vi "0xE7_Read_description_one_float_parameter.vi"(8 "error in":errorcluster, 10 "NumberFloatParam":i32 format="%0d", 11 "paramUnicornIn in":T2) -> (0 "error out":errorcluster, 1 "Param":T1, 2 "Тип/версия устройства":string, 3 "paramUnicornIn out 2":T2)   [LabVIEW 2017, in "LV_Unicorn.lvlib"]
uses:
  LV_Unicorn.lvlib
  Control/unicorn_Param.ctl
  Control/unicorn_conn.ctl
  Control/unicorn_JSON.ctl
  Control/unicorn_ParamInt.ctl
  Control/unicorn_Telemetry.ctl
  Control/unicorn_Table.ctl
  Control/unicorn_ParamFloat.ctl
  Control/unicorn_DescriptParam.ctl
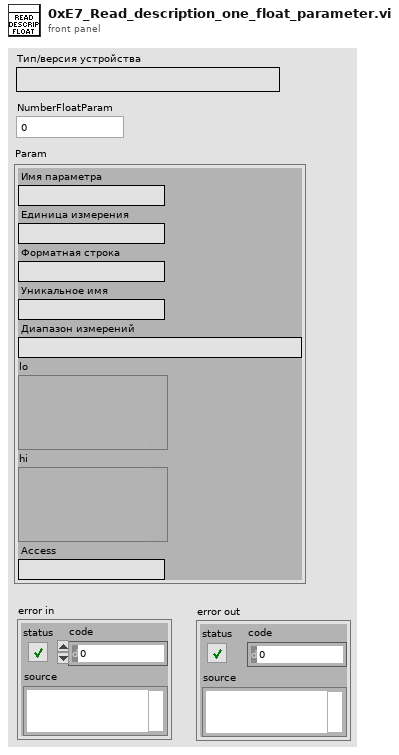
[diagram p1: front panel]
types:
  T1 = typedef "unicorn_DescriptParam.ctl" = cluster{"Имя параметра":string, "Единица измерения":string, "Форматная строка ":string, "Уникальное имя":string, "Диапазон измерений":string, "lo":variant, "hi":variant, "Access":string}
  T2 = typedef "LV_Unicorn.lvlib/unicorn_Param.ctl" = cluster{"conParam":T3, "Param":T4}
  T3 = typedef "LV_Unicorn.lvlib/unicorn_conn.ctl" = cluster{"ReadIntParam":bool, "ReadDescrParam":bool, "ReadFloatParam":bool, "debug":bool, "ReadJSON":bool, "IP_address":string, "N_attempts":i32, "type_con":enum16{"Serial", "TCP"}, "MB_address":i32, "VISA":refnum<visa-resource-name>, "connection ID":refnum<k5>, "nameDevices":string, "timeout":i32, "port":u16, "type_version":string, "baud_rate":u32, "VersionControl":bool, "TCP_conn":bool, "WindowSize":i32}
  T4 = typedef "LV_Unicorn.lvlib/unicorn_JSON.ctl" = cluster{"NumParam":cluster{"NTelem":i32, "NInt":i32, "NFloat":i32, "NTable":i32}, "ParamInt":T5, "Telemetry":T6, "Table":T7, "ParamFloat":T8}
  T5 = typedef "LV_Unicorn.lvlib/unicorn_ParamInt.ctl" = cluster{"ID":string, "Num":i32, "Name":string, "Type":string, "Enum":string, "Desc":string, "Unit":string, "Access":string, "FormatStr":string, "Min":i32, "Max":i32}[]
  T6 = typedef "LV_Unicorn.lvlib/unicorn_Telemetry.ctl" = cluster{"ID":string, "Num":i32, "Name":string, "Desc":string, "Unit":string, "FormatStr":string, "Min":i32, "Max":i32}[]
  T7 = typedef "LV_Unicorn.lvlib/unicorn_Table.ctl" = cluster{"Num":i32, "Access":string, "ColumnCount":i32, "NeedParamPrepare":bool, "Columns":cluster{"Column":i32, "Desc":string, "Name":string}[], "DataType":string, "FormatStr":string, "ID":string, "Name":string, "RowCount":i32, "Rows":cluster{"Desc":string, "ID":string, "Max":i32, "Min":i32, "Name":string, "Row":i32, "Unit":string}[], "Type":string}[]
  T8 = typedef "LV_Unicorn.lvlib/unicorn_ParamFloat.ctl" = cluster{"ID":string, "Num":i32, "Name":string, "Type":string, "Enum":string, "Desc":string, "Unit":string, "Access":string, "FormatStr":string, "Min":sgl, "Max":sgl}[]
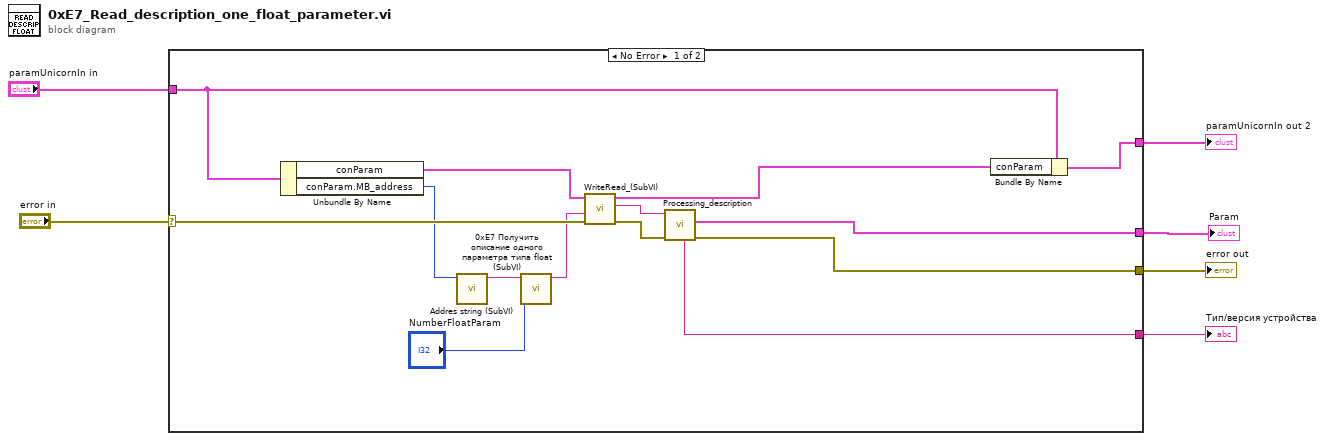
[diagram p0: block diagram]
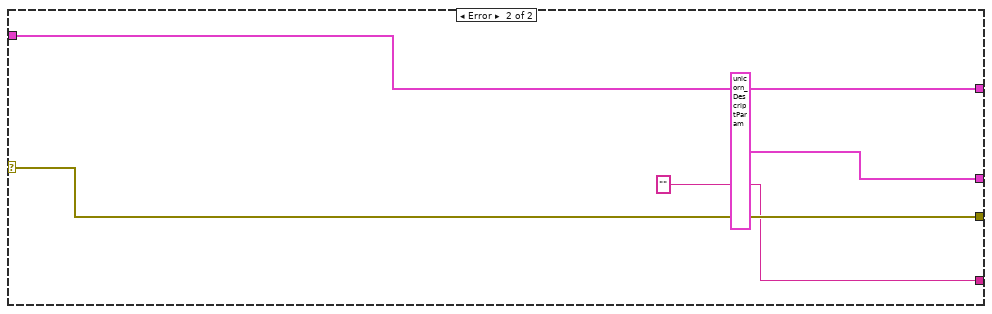
[diagram p2: hidden frame]
diagram:
  n1 = case shown="No Error" "error in" {
    selector: "error in" -> [w19 w24]
    tunnel: [w16 w24] -> w6
    tunnel: "paramUnicornIn in" -> [w11 w23]
    tunnel: [w13 w23] -> w4
    tunnel: [w15 T1 {"Имя параметра"="", "Единица измерения"="", "Форматная строка "="", "Уникальное имя"="", "Диапазон измерений"="", "lo"=variant, "hi"=variant, "Access"=""} ("Param")] -> w2
    tunnel: [w14 "" ("Ответ")] -> w1
    frame No Error {
      n2 = Unbundle By Name(w11) -> ("conParam"=w20:T3, "conParam.MB_address"=w10:i32)
      n3 = call "Addres string (SubVI).vi"("Адрес"=w10) -> ("String"=w9:string)  [unwired: 10 in]
      n4 = call "0xE7 Получить описание одного параметра типа float (SubVI).vi"("NumberFloatParam"="NumberFloatParam", "String in"=w9) -> ("String out"=w8:string)  [unwired: 9 in]
      n5 = call "WriteRead_(SubVI).vi"("error in"=w19, "Запрос"=w8, "ParamIn"=w20) -> ("error out"=w18:errorcluster, "Ответ"=w17:string, "ParamOut"=w12:T3)  [unwired: 4 in, 2 out]
      n6 = call "Processing_description.vi"("error in"=w18, "Ответ устройства"=w17) -> ("error out"=w16:errorcluster, "Param"=w15:T1, "Тип/версия устройства"=w14:string)  [unwired: 6 in, 1 out]
      n7 = Bundle By Name(cluster=w11, "conParam"=w12) -> (w13:T2)
    }
    frame Error {
    }
  }
  "error out" <- w6
  "paramUnicornIn out 2" <- w4
  "Param" <- w2
  "Тип/версия устройства" <- w1
